vi "Plotting.vi"() -> ()   [LabVIEW 2021]
panel:
  out "Thermometer":dbl(slide) scale=0.0..100.0
  out "Waveform Chart":dbl(graph)
  in  "Lower Temp Limit":dbl
  in  "Upper Temp Limit":dbl
  in  "stop":bool
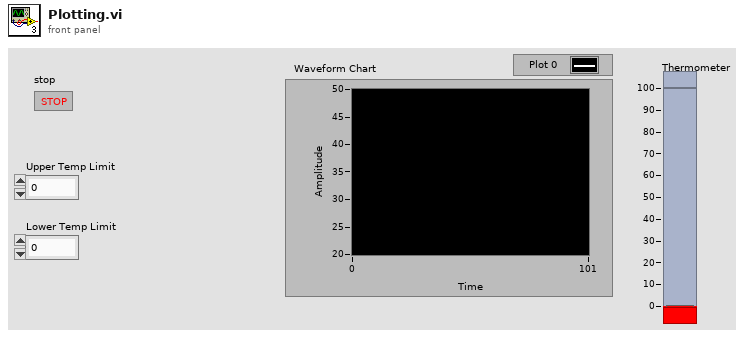
[diagram p1: front panel]
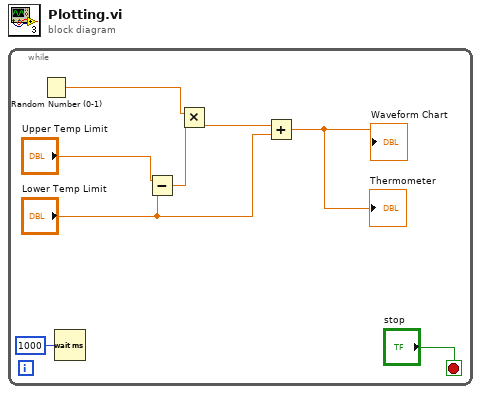
[diagram p0: block diagram]
diagram:
  n1 = while {
    stop <- "stop" stop-if-true
    n2 = Random Number (0-1)() -> (number: 0 to 1=w5:dbl)
    n3 = Wait (ms)(milliseconds to wait=u32 1000) -> ()  [unwired: 1 out]
    n4 = Subtract(x="Upper Temp Limit", y="Lower Temp Limit") -> (x-y=w3:dbl)
    n5 = Multiply(x=w5, y=w3) -> (x*y=w4:dbl)
    n6 = Add(x=w4, y="Lower Temp Limit") -> (x+y=→"Waveform Chart" →"Thermometer":dbl)
  }
